vi "GetNodeAttributeValue.vi"(8 "Error In":errorcluster, 10 "Attribute Name":string, 11 "Node In":refnum<k20>) -> (0 "Error Out":errorcluster, 2 "Value":string, 3 "Node Out":refnum<k20>)   [LabVIEW 2012, in "LV-Utilities.lvlib"]
uses:
  LV-Utilities.lvlib
  <resource>/objmgr/DOMUserDefRef.rc
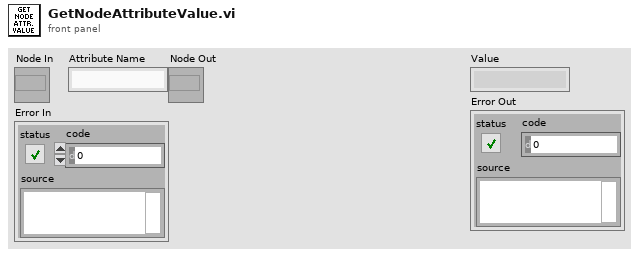
[diagram p1: front panel]
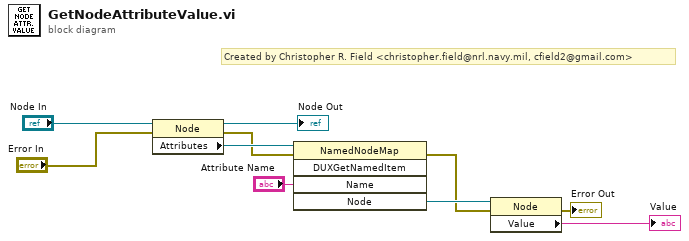
[diagram p0: block diagram]
diagram:
  # "Created by Christopher R. Field <christopher.field@nrl.navy.mil, cfield2@gmail.com>"
  n1 = property class="Node"(reference="Node In", error in="Error In") -> (reference out=→"Node Out":refnum<k20>, error out=w8:errorcluster, "Attributes"=w9:refnum<k20>)
  n2 = invoke class="NamedNodeMap" method="DUXGetNamedItem"(reference=w9, error in=w8, "Name"="Attribute Name") -> (error out=w4:errorcluster, "Node"=w5:refnum<k20>)  [unwired: 2 in, 3 out]
  n3 = property class="Node"(reference=w5, error in=w4) -> (error out=→"Error Out":errorcluster, "Value"=→"Value":string)  [unwired: 1 out]
